vi "Get Vector Magnitude.vi"(8 "error in":errorcluster, 11 "PVector in":refnum<class "PVector.lvclass">) -> (0 "error out":errorcluster, 2 "Mag(V)":dbl, 3 "PVector out":refnum<class "PVector.lvclass">)   [LabVIEW 2016, in "PVector.lvclass"]
doc: "Returns vector V magnitude ||V||"
uses:
  PVector.lvclass
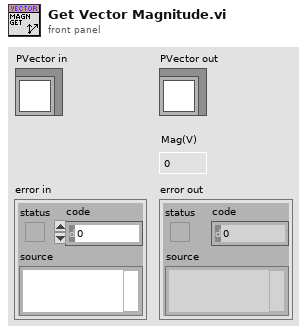
[diagram p1: front panel]
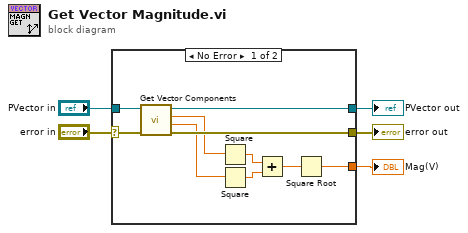
[diagram p0: block diagram]
diagram:
  n1 = case shown="No Error" "error in" {
    selector: "error in" -> [w14 w17]
    tunnel: [w13 w17] -> w4
    tunnel: [w12 w16] -> w2
    tunnel: "PVector in" -> [w15 w16]
    tunnel: [w6 _] -> w1
    frame No Error {
      n2 = call "Get Vector Components.vi"("error in"=w14, "PVector in"=w15) -> ("error out"=w13:errorcluster, "Y"=w10:dbl, "X"=w11:dbl, "PVector out"=w12:refnum<class "PVector.lvclass">)  [unwired: 6 in]
      n3 = Square(x=w11) -> (x^2=w9:dbl)
      n4 = Square(x=w10) -> (x^2=w8:dbl)
      n5 = Add(x=w9, y=w8) -> (x+y=w7:dbl)
      n6 = Square Root(x=w7) -> (sqrt(x)=w6:dbl)
    }
    frame Error {
    }
  }
  "error out" <- w4
  "PVector out" <- w2
  "Mag(V)" <- w1
